vi "Set Rotation.vi"(8 "error in":errorcluster, 11 "IMG_SRC in":refnum<class "IMG_SRC.lvclass">) -> (0 "error out":errorcluster, 2 "Supported?":bool, 3 "IMG_SRC out":refnum<class "IMG_SRC.lvclass">)   [LabVIEW 2018, in "IMG_SRC.lvlib" / "IMG_SRC.lvclass"]
uses:
  IMG_SRC.lvclass
  IMG_SRC.lvclass/IMG_SRC.ctl
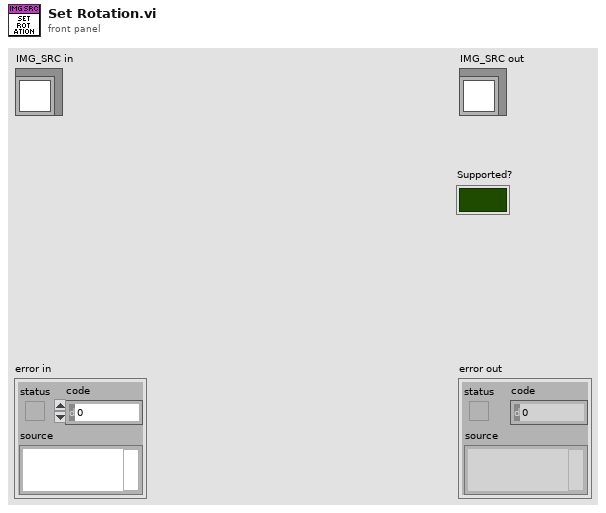
[diagram p1: front panel]
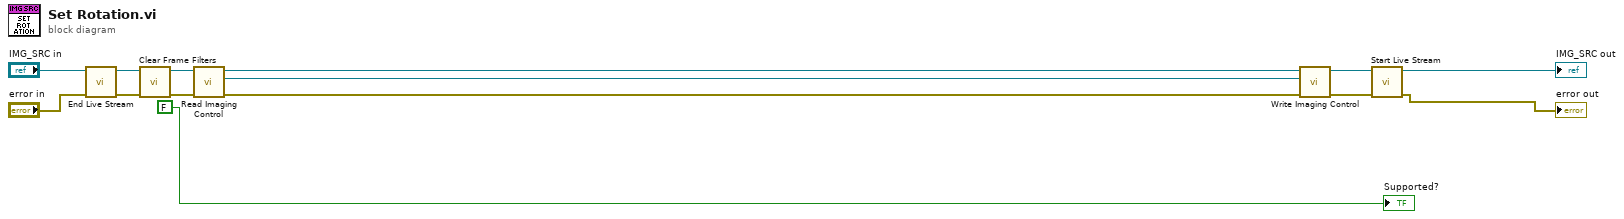
[diagram p0: block diagram]
diagram:
  n1 = call "End Live Stream.vi"("error in"="error in", "IMG_SRC in"="IMG_SRC in") -> ("error out"=w3:errorcluster, "IMG_SRC out"=w4:refnum<class "IMG_SRC.lvclass">)  [unwired: 8 in]
  n2 = call "Clear Frame Filters.vi"("error in"=w3, "IMG_SRC in"=w4) -> ("error out"=w2:errorcluster, "IMG_SRC out"=w1:refnum<class "IMG_SRC.lvclass">)  [unwired: 8 in]
  n3 = call "Read Imaging Control.vi"("error in (no error)"=w2, "IMG_SRC in"=w1) -> ("error out"=w13:errorcluster, "Imaging Control"=w12:refnum<k7>, "IMG_SRC out"=w14:refnum<class "IMG_SRC.lvclass">)  [unwired: 7 in]
  n4 = call "Write Imaging Control.vi"("error in (no error)"=w13, "Imaging Control"=w12, "IMG_SRC in"=w14) -> ("error out"=w7:errorcluster, "IMG_SRC out"=w8:refnum<class "IMG_SRC.lvclass">)  [unwired: 7 in]
  n5 = call "Start Live Stream.vi"("error in"=w7, "IMG_SRC in"=w8) -> ("error out"=→"error out":errorcluster, "IMG_SRC out"=→"IMG_SRC out":refnum<class "IMG_SRC.lvclass">)  [unwired: 8 in]
  "Supported?" <- FALSE
